vi "Robot Main.vi"   [LabVIEW 2013]
doc: "This VI imlements the framework and scheduler for your robotics program. It should not be necessary to modify the framework. You are expected to add your code to the VIs called from Robot Main, the ones located in the Team Code within the project."
panel:
  # "2014 ÜberCode"
  # "Version 1.1_Fri: 3-14-2014"
  # "Todo"
  # "Controls"
  # "PWM"
  # "DIO"
  # "Relay"
  # "Analog"
  # "Solenoid"
  # "- Clean Up Code\n- Empty old code out\n- Prepare Vision\n- Implement new systems with joystick buttons/axis\n-Make loops communicate to eachother\n-Add working auto distance for shooting\n-Finish (un-tuned) code\n-Dashboard comms\n-Custom Dashboard Project\n-use hat switch?\n-tune for suffield"
  # "Joystick 1 (Logitech Attack 3)\nX Axis: Arcade Drive \nY Axis: Arcade Drive \nZ Axis:\nButton 1: Hold Position Toggle\nButton 2:\nButton 3:\nButton 4:\nButton 5: \nButton 6: \nButton 7: Shift High\nButton 8: Toggle Vision\nButton 9: \nButton 10: Go To Shoot Location\nButton 11: Disable Vision & GoTo DC\nButton 12: Shift Low"
  # "Joystick 2 (Logitech Extreme 3D)\nX Axis: \nY Axis: Belts Manual Override/DC \nZ Axis: Tune Belt Speed\nButton 1: \nButton 2: \nButton 3: Null state mach and belts\nButton 4: \nButton 5: Belts Driver Control\nButton 6: Belts Manual Override\nButton 7: \nButton 8: \nButton 9: Cancel Pickup Mode\nButton 10: \nButton 11: Pickup (For Passing)\nButton 12: Pass"
  # "Joystick 3 (Logitech Extreme 3D)\nX Axis: \nY Axis: Pickup Arm Manual Overide\nZ Axis: Tune Pickup Arm Pickup Height\nButton 1: Shoot\nButton 2: Load\nButton 3: null arm\nButton 4: \nButton 5: Arm Driver Control\nButton 6: Arm Manual Override\nButton 7: Home Arm\nButton 8: Manual Shoot\nButton 9: Shooter Position Toggle\nButton 10: Latch Position Toggle\nButton 11: Cancel Load Mode\nButton 12:"
  # "1 a): Right Front Drive\n1 b): Right Rear Drive\n2 a): Left Front Drive\n2 b): Left Rear Drive\n3 a): Right Pickup Motor\n3 b): Left Pickup Motor\n     4: Pickup Belt\n     5:  \n     6: \n     7: \n     8: \n     9: \n   10:"
  # "1: Right Drive Encoder A\n  2: Right Drive Encoder B\n  3: Left Drive Encoder A  \n  4: Left Drive Encoder B\n  5: Pickup Motor Encoder A\n  6: Pickup Motor Encoder B\n  7: Shooter Magnetic Sensor R-Up\n  8: Shooter Magnetic Sensor R-Down\n  9: 2 Ball Auto Toggle Switch\n10: \n11: \n12: Holding Light Sensor\n13: \n14: Pneumatic Pressure Switch"
  # "1: Compressor Spike\n2:\n3:\n4:\n5:\n6:\n7:\n8:"
  # "1:\n2:\n3:\n4:\n5:\n6:\n7:\n8:"
  # "1: Latch A\n2: Latch B\n3: Shooter A\n4: Shooter B\n5: Shifter A\n6: Shifter B\n7:\n8:"
  # "Hat Switch Up: Increment Arm Setpoint\nHat Switch Down: Decrement Arm Setpoint"
  # "Revision History"
  # "-removed unnecessary support code VIs\n-added latch engaged sensor\n-constants needing tuning changed to controls\n-made goto shoot change to hold position when done\n0.5\n-removed 3 of the 4 piston sensors :'(\n-shooter piston code compensates for ^\n-edited build custom dashboard data vi\n-updated arm saftey to match dashboard\n0.6\n-Misc. improvements\n0.7\n-Added more magnetic piston sensors :)\n-Edited code to compensate for ^\n-changed axis 3 to 4 because of new joysticks\n-fixed bug in belt code\n-changed pickup arm hold position code\n-removed unnecessary support code VIs\n-added latch engaged sensor\n-changed joystick 1 layout\n-updated begin and finish VIs\n-latch leaves shoot after shoots\n-updated shoot safely.vi\n-incorporated error filters on axes\n0.8\n-changed home arm button\n-added cancel commands to teleop code\n-removed latch sensor\n-renamed lock back to latch\n-added manual shoot (dry fire) to latch\n-changed teleop for cancels (improved)\n-latch only stays in an actuation state for one iteration\n0.9\n-adapted latch teleop manual override to shooter control cancel code\n-no safe dry fire\n-adapt teleop to no safe dry fire"
  # "-put can shoot safely FG into load state machine\n-that is reset in shoot\n-removed joysticks from dashboard, along with the substate manager fg\n-fixed state machine load to keep saying cock, retract, latch, or unlatch until it is confirmed\n-adapted all state machines to use the refnum FG\n-finished cancel state machine\n-non drive related teleop loops feedback nodes default to null\n-changed teleop to send commands to loop 1\n-finish vi uncocks shooter\n-changed load to retract shooter\n-changed canceling code to use joystick instead of previous command\n-fg for canceling is overriten at each new use in pickup and load, and at the end of\ncancel\n-put can shoot safely FG into load state machine\n-that is reset in shoot\n-removed joysticks from dashboard, along with the substate manager fg\n-fixed state machine load to keep saying cock, retract, latch, or unlatch until it is confirmed\n-adapted all state machines to use the refnum FG\n-fixed cancel to work with different load logic\n-remove now obsolete cancel fg\n-fixed up cancel state machine entirely\n-cleaned up dashboard code a bit\n-safe shooting\n-update devref database fg name and implimentation in all state machines\n-arm rate PID"
  # "0.1\n-Blank(ish) structure\n0.2\n-Cleaned out old game-specific code\n-Updated VIs\n-Added vision/changed vision\n-finished distance\n0.3\n-modified teleop and structure\n-basic teleop complete, auto ready for setup\n-goto shoot vi added\n-configured begin vi\n-worked on structure/arm vi\n0.4\n-edited goto shoot vi\n-revised vision calculating vi\n-changed joystick layouts\n-no longer use holding sensor\n-arm code done (untuned)\n-belt code done (untuned)\n-shooter code done (untuned)\n-go to shoot code done (untuned)\n-vision done (untuned)\n-constants needing tuning changed to controls\n-made goto shoot change to hold position when done\n0.5\n-removed 3 of the 4 piston sensors :'(\n-shooter piston code compensates for ^\n-edited build custom dashboard data vi\n-updated arm saftey to match dashboard\n0.6\n-Misc. improvements\n0.7\n-Added more magnetic piston sensors :)\n-Edited code to compensate for ^\n-changed axis 3 to 4 because of new joysticks\n-fixed bug in belt code\n-changed pickup arm hold position code"
  # "-adapt teleop to no safe dry fire\n-changed belt and arm code to have one setpoint and have a hold sensor\n-minor bugfixes\n-updated begin\n-arm encoder distance per count calculated\n1.0\n-added all state machines\n-state machines use U8 integers\n-properly implimented state machines-added FGs for arm and belts\n-tuner for belts\n-tuner for arm setpoint\n-PID for arm tuned\n-found setpoints for arm\n-safety for arm done\n-removed old loop 4\n-pneumatics in one loop\n-pneumatics became loop 4\n-changed pneumatics type def\n-single use substate fg\n-made pneumatics able to be set by the single use substate fg (teleop)\n-pneumatics loop only stays in a set state for 1 iteration (teleop code)\n-put exit in true constants on all state fgs in state machines-state machines report that they are done\n-fg for canceling efficiently\n-finished cancel state machine\n-non drive related teleop loops feedback nodes default to null\n-changed teleop to send commands to loop 1\n-finish vi uncocks shooter\n-changed load to retract shooter\n-changed canceling code to use joystick instead of previous command\n-fg for canceling is overriten at each new use in pickup and load, and at the end of\ncancel"
  # "-all state machines wait for actions to finish before continuing\n-renamed shooter loop to a more descriptive, accurate name\n-timeout vi and timeout error fg\n-js1 is a logitech extreme 3d again..\n-fixed timeout fg\n-reduce magic number syndrome in master loop functions\n-disabled rate pid\n-changed a typedef to say joystick z instead of tune speed\n-incorporated auto drive\n-made auto state machine\n-worked on auto state for master loop\n-updated state machines\n-re-did auto state machine\n-small auto change\n-major work done on auto state machine, states 0-7 out of 10 done\n-finished auto state machine\n-minor bugfixes in auto loop\n-purged load state mach of auto mode code\n-put updated vision begin and processor from vision practice project\n-re-did most of autonomous vi-it reads data from states fg for loops 2-4. 0-1 still use pre-coded commands\n-bugfixes in auto and load state machines\n-started arm dc vi\n-fixed cancel arm during load exception\n-worked on pickup arm driver control\n-arm driver control setpoint vi works in theroy...\n-tuned arm constants in a seperate vi and moved logic back into this\n-minor main ctrl cleanup\n-deleted unnecessary vis\n-added 2 ball switch\n-updated finish.vi for 2 ball close\n-increased arm dc effeciency"
  # "-all state machines use constants for transitions (I think)\n-bugfixes\n-timeout bi and error log fg\n-sped up code\n-end case for pneuatics\n-timeouts reset\n-network tables dashboard\n-milisecond timestamp to error logger\n-all state machines work\n-pre-groton edits\n-groton day one, removed timeout code\n-groton day 2\n-cleaned up dev ref data base\n-cleaned up messy groton code\n-manual override arm overrides safeties\n-manual override pistons\n-pass adapts for failed pass\n-re-incorporated arm rate pid\n-minor auto changes\n-touched up passing\n-minor changes to rate arm pid\n-incorporated test code\n-arm rate and distance pids are ready\n-auto drive uses rate and distance pids\n-auto loop 0 can go back to normal auto functionality"
  # "-"
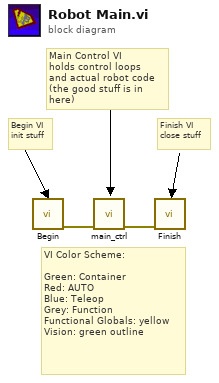
[diagram p0: block diagram]
diagram:
  # "Finish VI\nclose stuff"
  # "Main Control VI\nholds control loops\nand actual robot code\n(the good stuff is in here)"
  # "Begin VI\ninit stuff"
  # "VI Color Scheme:\n\nGreen: Container\nRed: AUTO\nBlue: Teleop\nGrey: Function\nFunctional Globals: yellow\nVision: green outline"
  n1 = call "Begin.vi"() -> ("error out"=w2:errorcluster)  [unwired: 1 in, 10 out]
  n2 = call "main_ctrl.vi"("error in"=w2) -> ("error out"=w1:errorcluster)  [unwired: 10 in]
  n3 = call "Finish.vi"("error in"=w1) -> ()  [unwired: 7 in]
